vi "Write_Path-to-logfile.vi"(8 "error in (no error)":errorcluster, 10 "Path to logfile":path, 11 "StatusLog in":refnum<class "StatusLog.lvclass">) -> (0 "error out":errorcluster, 3 "StatusLog out":refnum<class "StatusLog.lvclass">)   [LabVIEW 2018, in "StatusLog.lvclass"]
uses:
  StatusLog.lvclass
  StatusLog.lvclass/StatusLog.ctl
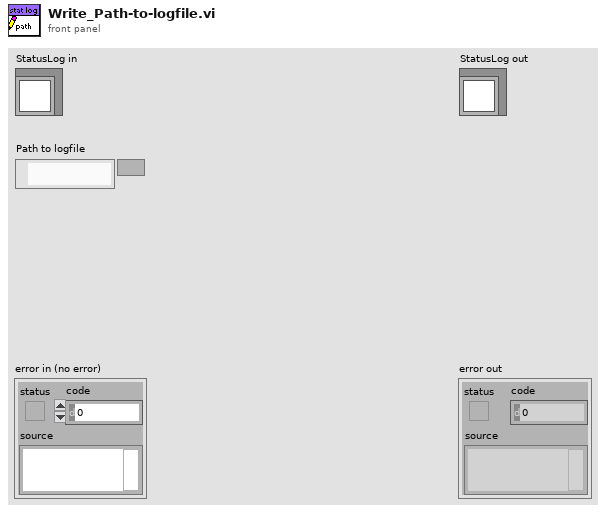
[diagram p1: front panel]
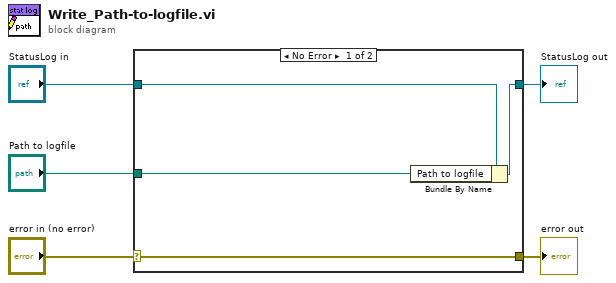
[diagram p0: block diagram]
diagram:
  n1 = case shown="No Error" "error in (no error)" {
    selector: "error in (no error)" -> [w9 w10]
    tunnel: [w9 w10] -> w4
    tunnel: [w7 w11] -> w2
    tunnel: "StatusLog in" -> [w8 w11]
    tunnel: "Path to logfile" -> [w6 _]
    frame No Error {
      n2 = Bundle By Name(cluster=w8, "Path to logfile"=w6) -> (w7:refnum<class "StatusLog.lvclass">)
    }
    frame Error {
    }
  }
  "error out" <- w4
  "StatusLog out" <- w2
